vi "RunHotLot.vi"() -> ()   [LabVIEW 2012]
uses:
  <vilib>/addons/database/Connection.llb/DB Tools Open Connec (Path).vi
  <vilib>/addons/database/NI_Database_API.lvlib
panel:
  out "data 2":string
  out "Array 2":string[][](array[string])
  out "Array":string[][](array[string])
  out "data":string
  in  "Cluster":T1
  out "error out":errorcluster
  out "String":string
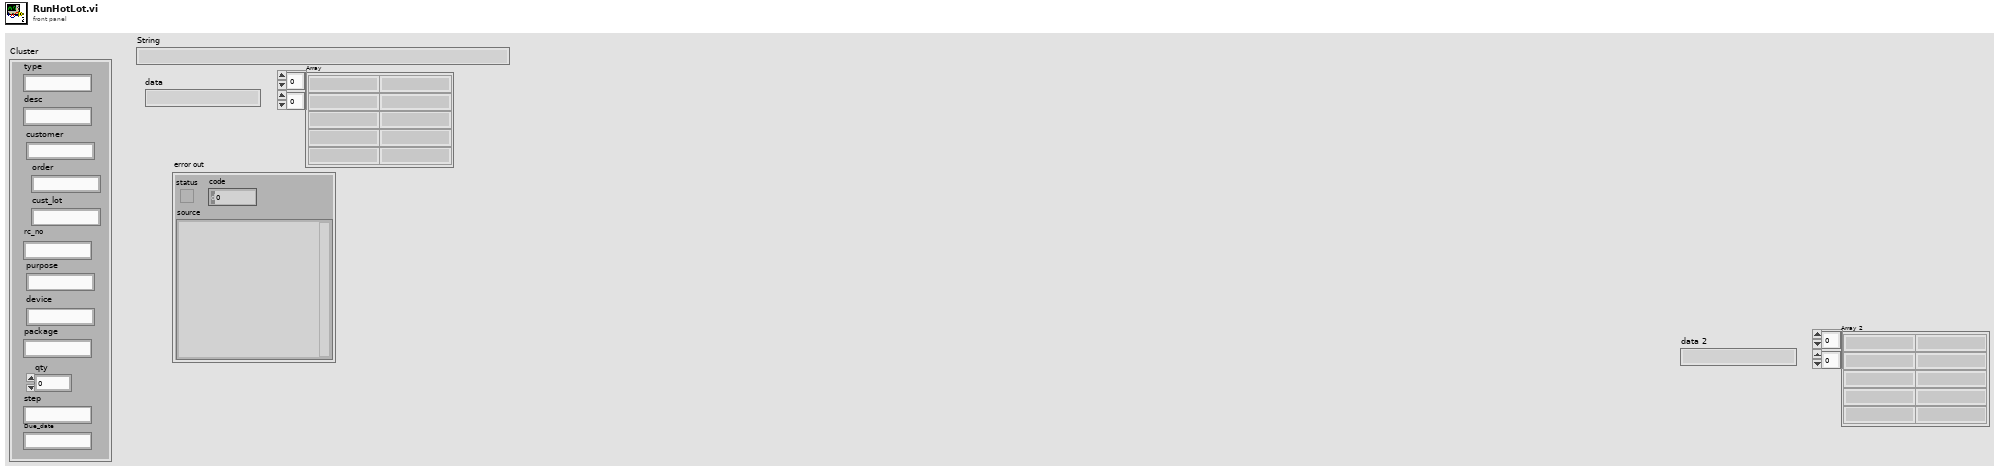
[diagram p1: front panel]
types:
  T1 = cluster{"type":string, "desc":string, "customer":string, "order":string, "cust_lot":string, "rc_no":string, "purpose":string, "device":string, "package":string, "qty":dbl, "step":string, "Due_date":string}
  T2 = typedef "NI_Database_API.lvlib/Conn ObjectReference.ctl" = refnum<k1>
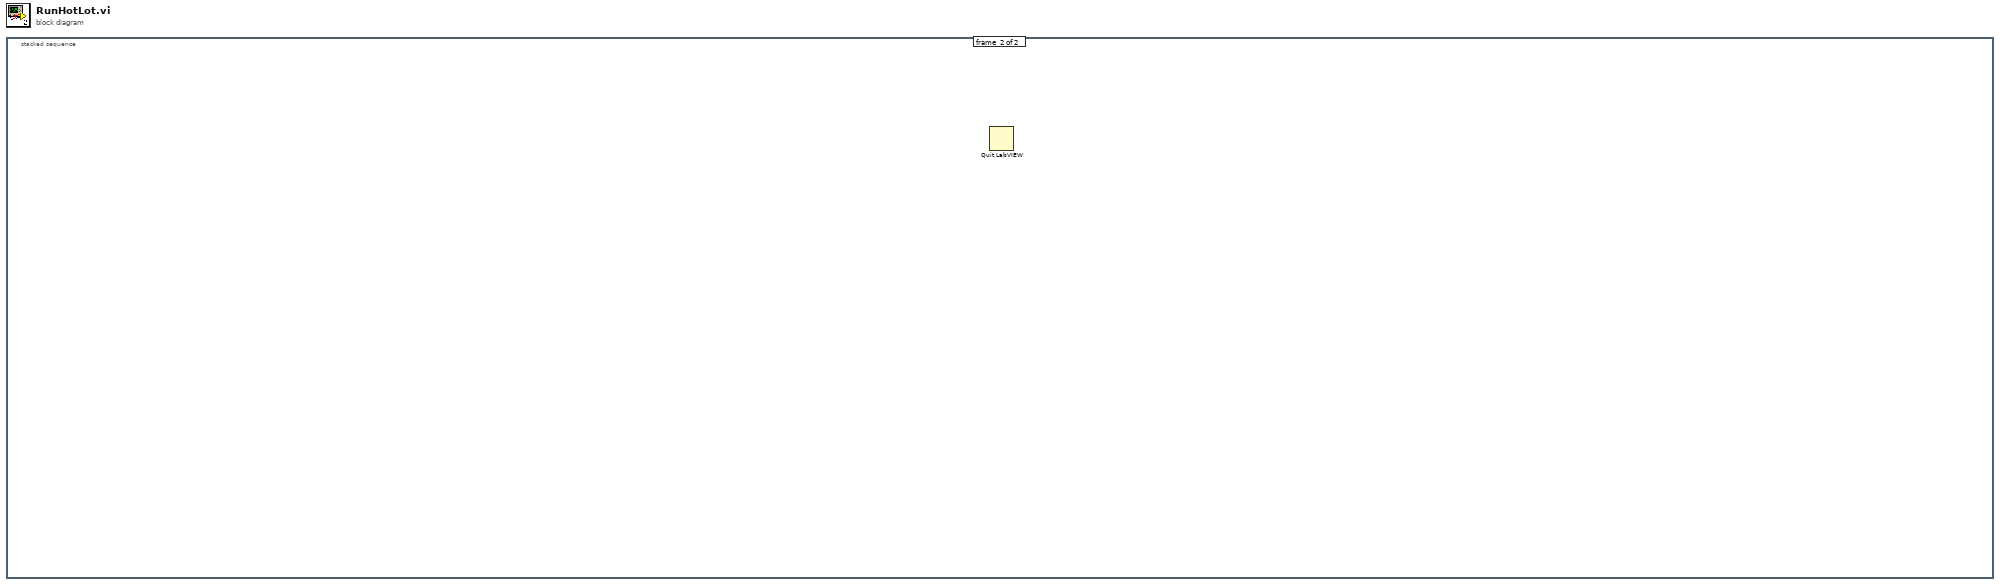
[diagram p0: block diagram]
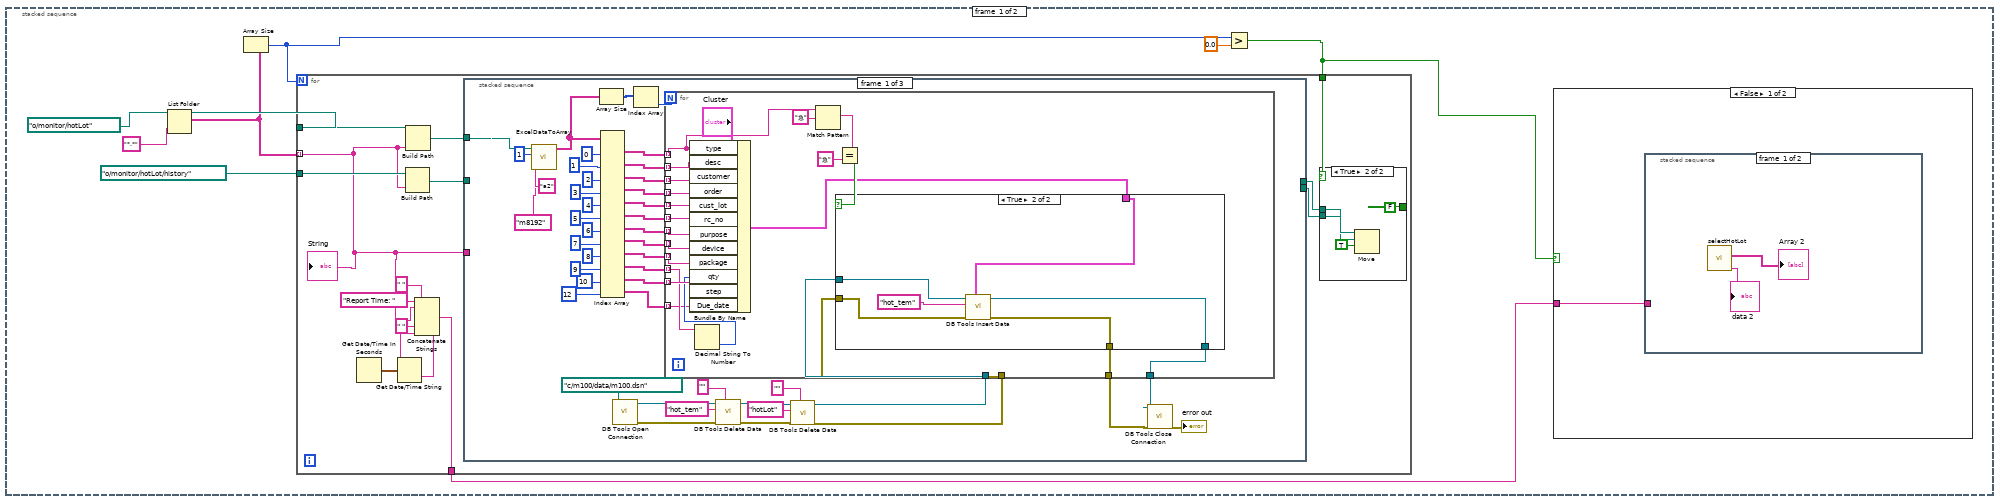
[diagram p2: hidden frame]
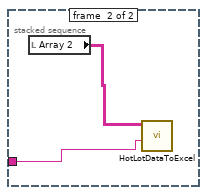
[diagram p3: hidden frame]
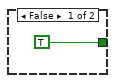
[diagram p5: hidden frame]
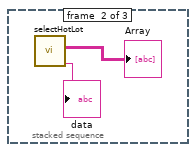
[diagram p7: hidden frame]
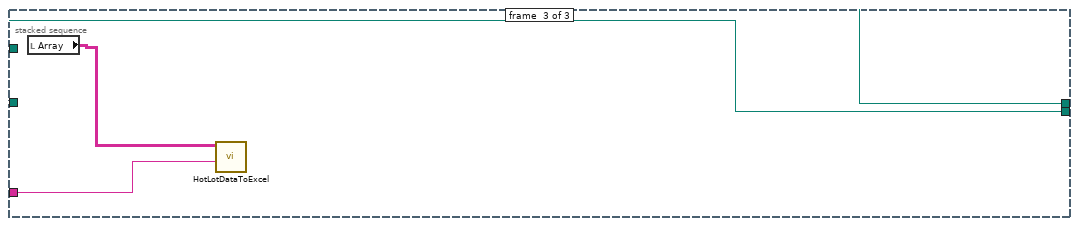
[diagram p8: hidden frame]
diagram:
  n1 = stacked-sequence {
    frame #0 {
      n2 = List Folder(path=path "o:/monitor/hotLot", pattern="*.*") -> (path out=w7:path, filenames=w2:string[])  [unwired: 2 in, 2 out]
      n3 = Array Size(array=w2) -> (size(s)=w1:i32)
      n4 = Greater?(x=w1, y=0.0) -> (0:w4:bool)
      n5 = for {
        N: w1 -> [_]
        tunnel: w7 -> [w29]
        tunnel: path "o:/monitor/hotLot/history" ("base path") -> [w27]
        tunnel: w4 -> [w23]
        tunnel: [w16] -> w3
        tunnel: w2 -> [w15] mode=indexing
        n6 = Get Date/Time In Seconds() -> (seconds since 1Jan1904=w22:timestamp)
        n7 = Get Date/Time String(seconds (now)=w22) -> (date string=w20:string, time string=w18:string)  [unwired: 2 in]
        n8 = Build Path(base path=w27, name or relative path=w15) -> (appended path=w26:path)
        n9 = Build Path(base path=w29, name or relative path=w15) -> (appended path=w28:path)
        n10 = Concatenate Strings("Report Time: " ("string"), w20, " " ("string"), w18, " " ("string"), w15) -> (w16:string)
        n11 = stacked-sequence {
          tunnel: w28 -> [w47 _ w116]
          tunnel: w26 -> [_ _ w115]
          tunnel: [_ _ w116] -> w25
          tunnel: [_ _ w115] -> w24
          tunnel: w15 -> [_ _ w113]
          frame #0 {
            n12 = call "ExcelDataToArray.vi"("end cell"="m8192", "start cell"="a2", "sheet#"=1, "path"=w47) -> ("data"=w71:string[][])  [unwired: 6 in, 1 out]
            n13 = Array Size(array=w71) -> (size(s)=w75:i32[])
            n14 = Index Array(array=w71, index (col) #1=0 ("disabled index (col)"), index (col) #2=1 ("index (col)"), index (col) #3=2 ("index (col)"), index (col) #4=3 ("index (col)"), index (col) #5=4 ("index (col)"), index (col) #6=5 ("index (col)"), index (col) #7=6 ("index (col)"), index (col) #8=7 ("index (col)"), index (col) #9=8 ("index (col)"), index (col) #10=9 ("index (col)"), index (col) #11=10 ("index (col)"), index (col) #12=12 ("index (col)")) -> (element #1=w60:string[], element #2=w59:string[], element #3=w58:string[], element #4=w57:string[], element #5=w56:string[], element #6=w55:string[], element #7=w54:string[], element #8=w53:string[], element #9=w52:string[], element #10=w51:string[], element #11=w50:string[], element #12=w45:string[])  [unwired: 12 in]
            n15 = call-poly <vilib>:"DB Tools Open Connection.vi"("connection information"=path "c:/m100/data/m100.dsn") -> ("error out"=w43:errorcluster, "connection reference"=w44:T2)  [unwired: 7 in]
            n16 = Index Array(array=w75) -> (element=w74:i32)  [unwired: 1 in]
            n17 = call <vilib>:"DB Tools Delete Data.vi"("condition"="", "error in (no error)"=w43, "table"="hot_tem", "connection reference"=w44) -> ("error out"=w41:errorcluster, "connection reference out"=w42:T2)  [unwired: 6 in]
            n18 = call <vilib>:"DB Tools Delete Data.vi"("condition"="", "error in (no error)"=w41, "table"="hotLot", "connection reference"=w42) -> ("error out"=w39:errorcluster, "connection reference out"=w40:T2)  [unwired: 6 in]
            n19 = for {
              N: w74 -> [_]
              tunnel: w60 -> [w82] mode=indexing
              tunnel: w59 -> [w100] mode=indexing
              tunnel: w58 -> [w99] mode=indexing
              tunnel: w57 -> [w98] mode=indexing
              tunnel: w56 -> [w97] mode=indexing
              tunnel: w55 -> [w86] mode=indexing
              tunnel: w54 -> [w93] mode=indexing
              tunnel: w53 -> [w94] mode=indexing
              tunnel: w52 -> [w95] mode=indexing
              tunnel: w51 -> [w88] mode=indexing
              tunnel: w50 -> [w96] mode=indexing
              tunnel: w40 -> [w90]
              tunnel: w39 -> [w89]
              tunnel: [w84] -> w49
              tunnel: [w85] -> w48
              tunnel: w45 -> [w83] mode=indexing
              n20 = Decimal String To Number(string=w88) -> (number=w87:i32)  [unwired: 2 in, 1 out]
              n21 = Bundle By Name(cluster="Cluster", "type"=w82, "desc"=w100, "customer"=w99, "order"=w98, "cust_lot"=w97, "rc_no"=w86, "purpose"=w93, "device"=w94, "package"=w95, "qty"=w87, "step"=w96, "Due_date"=w83) -> (w91:T1)
              n22 = Match Pattern(string=w82, regular expression="急") -> (match substring=w80:string)  [unwired: 1 in, 3 out]
              n23 = Equal?(x=w80, y="急") -> (x = y?=w92:bool)
              n24 = case shown="True" w92 {
                tunnel: w91 -> [_ w105]
                tunnel: w90 -> [w103 w109]
                tunnel: w89 -> [w104 w108]
                tunnel: [w104 w106] -> w85
                tunnel: [w103 w107] -> w84
                frame False {
                }
                frame True {
                  n25 = call <vilib>:"DB Tools Insert Data.vi"("data"=w105, "error in (no error)"=w108, "table"="hot_tem", "connection reference"=w109) -> ("error out"=w106:errorcluster, "connection reference out"=w107:T2)  [unwired: 6 in]
                }
              }
            }
            n26 = call <vilib>:"DB Tools Close Connection.vi"("error in (no error)"=w48, "connection reference"=w49) -> ("error out"=→"error out":errorcluster)  [unwired: 5 in]
          }
          frame #1 {
            n27 = call "selectHotLot.vi"() -> ("data"=→"data":string, "Array"=→"Array":string[][])  [unwired: 10 in]
          }
          frame #2 {
            n28 = local read "Array"() -> (w114:string[][])
            n29 = call "HotLotDataToExcel.vi"("Header"=w113, "data"=w114) -> ()  [unwired: 10 in]
          }
        }
        n30 = case shown="True" w23 {
          tunnel: w25 -> [_ w34]
          tunnel: w24 -> [_ w33]
          tunnel: [TRUE FALSE] -> _
          frame False {
          }
          frame True {
            n31 = Move(source path=w34, 9:TRUE ("overwrite (F)"), 10:w33) -> ()  [unwired: 2 in, 3 out]
          }
        }
        "String" <- w15
      }
      n32 = case shown="False" w4 {
        tunnel: w3 -> [w10 _]
        frame False {
          n33 = stacked-sequence {
            tunnel: w10 -> [_ w13]
            frame #0 {
              n34 = call "selectHotLot.vi"() -> ("data"=→"data 2":string, "Array"=→"Array 2":string[][])  [unwired: 10 in]
            }
            frame #1 {
              n35 = local read "Array 2"() -> (w14:string[][])
              n36 = call "HotLotDataToExcel.vi"("Header"=w13, "data"=w14) -> ()  [unwired: 10 in]
            }
          }
        }
        frame True {
        }
      }
    }
    frame #1 {
      n37 = Quit LabVIEW() -> ()  [unwired: 1 in]
    }
  }
